vi "Algo test.vi"() -> ()   [LabVIEW 2017]
uses:
  <vilib>/vision/Image Controls.llb/IMAQ Image.ctl
  File/Control/Folder Format.ctl
  File/Control/File Format.ctl
  File/Control/Parent path.ctl
  Toolbox/Control/CVT Action.ctl
  Toolbox/Control/CVT name.vi
  SubVI/File/Section and key name.vi
  <vilib>/vision/NI_Vision_Development_Module.lvlib
  <vilib>/vision/driver/NI_Vision_Acquisition_Software.lvlib
  <vilib>/userdefined/High Color/IMAQdx.ctl
  Toolbox/Toolbox.lvlib
  File/File.lvlib
panel:
  out "Excel copy_Gap inv":sgl[](array[numeric])
  out "Excel copy_Ering inv":dbl[](array[numeric])
  out "Excel copy_Gap":sgl[](array[numeric])
  out "Excel copy_Ering":dbl[](array[numeric])
  out "ERing 4":sgl[](array[numeric]) format="%.3g"
  out "ERing 3":sgl[](array[numeric]) format="%.3g"
  out "ERing 2":sgl[](array[numeric]) format="%.3g"
  out "ERing 1":sgl[](array[numeric]) format="%.3g"
  out "Row1":sgl[](array[numeric]) format="%.3g"
  out "Row2":sgl[](array[numeric]) format="%#.3g"
  out "Row3":sgl[](array[numeric]) format="%#.3g"
  out "Row4":sgl[](array[numeric]) format="%.3g"
  out "Row Match":bool[](array[boolean])
  out "Row time":u32[](array[numeric])
  in  "File Path 2":path
  out "Image":T1(plugin-control)
  out "error out":errorcluster
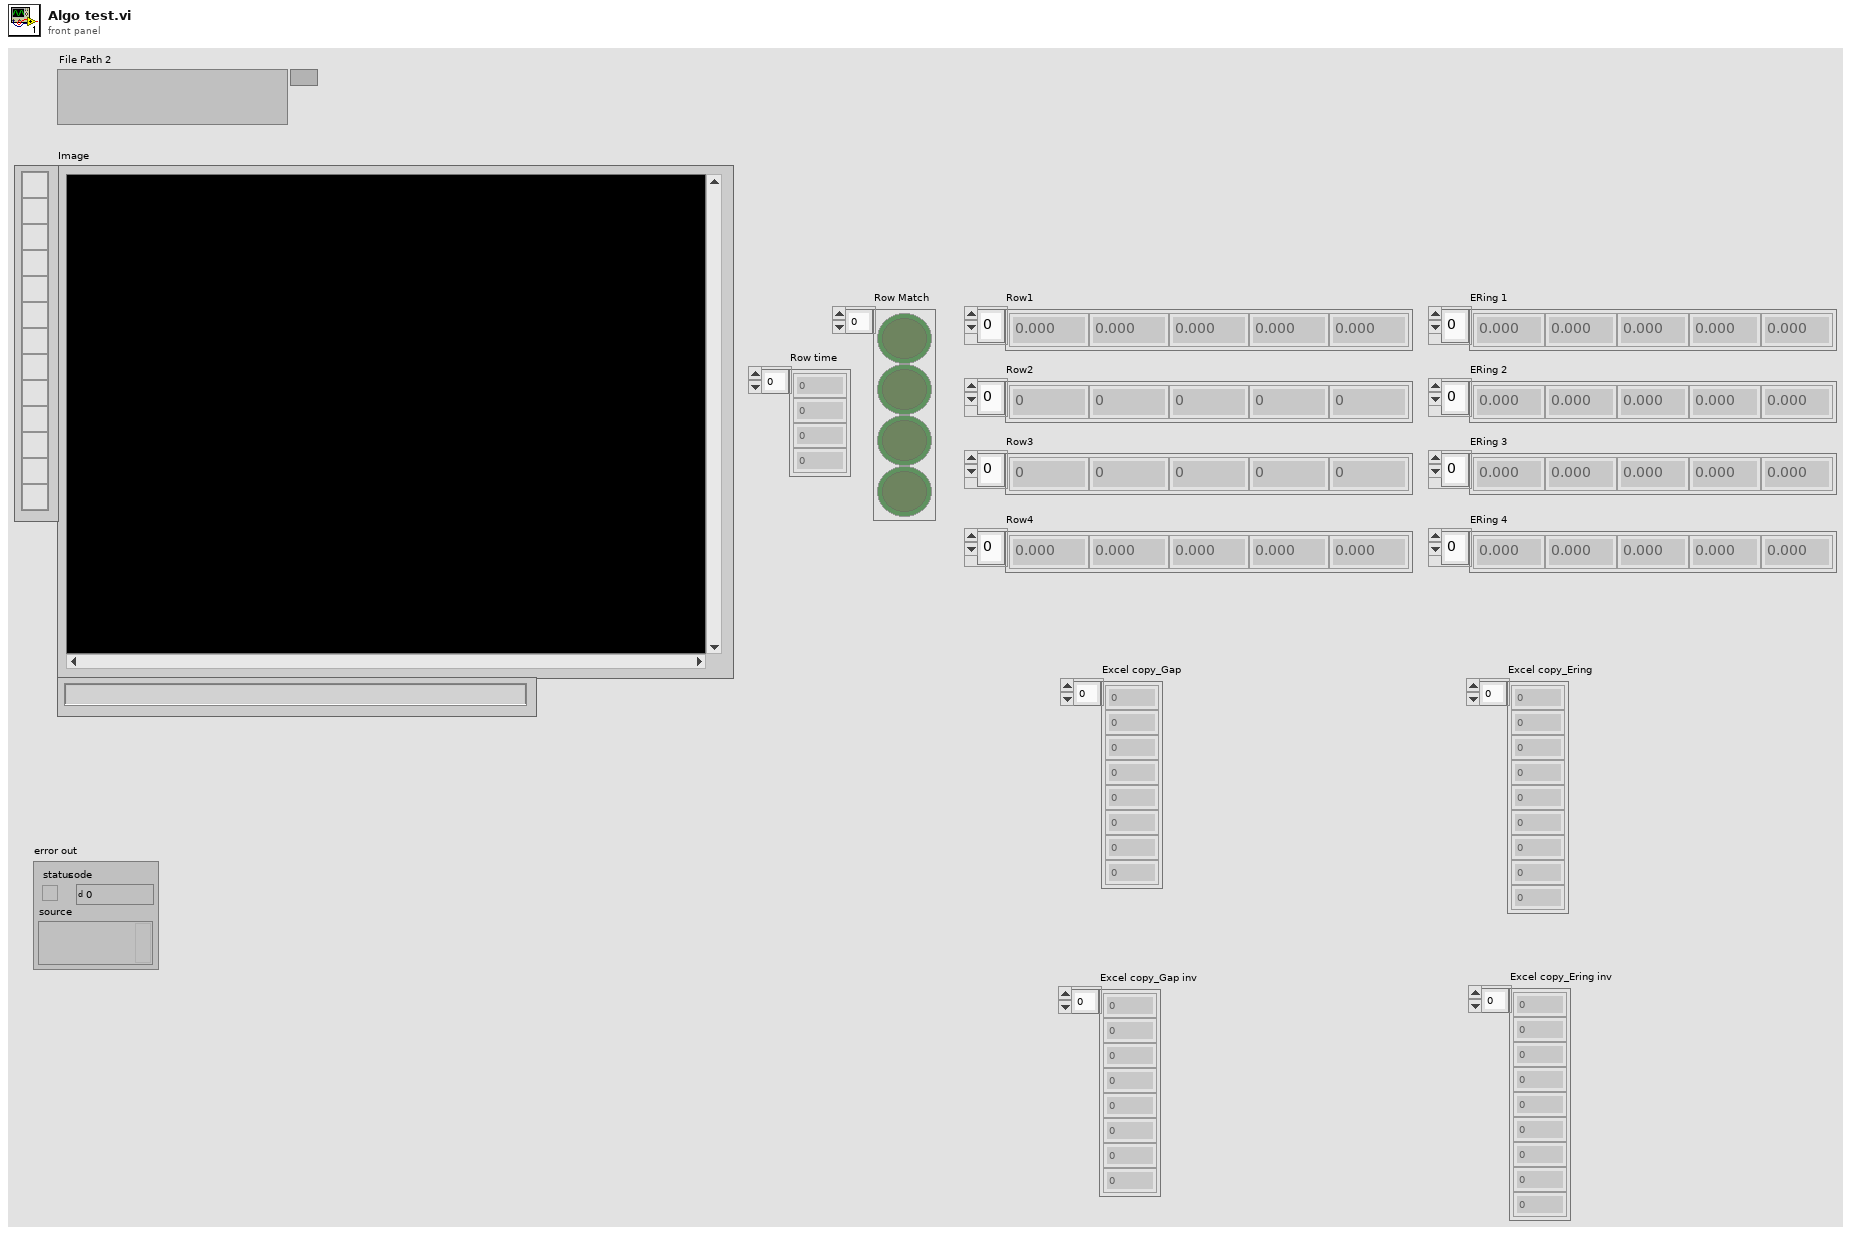
[diagram p1: front panel]
types:
  T1 = typedef "IMAQ Image.ctl" = refnum<image>
  T2 = cluster{"State":string, "snap Image":T1, "Template":T1, "Calibration":T1, "Row1 result":cluster{"Fitted Circle Ering":cluster{"Center (Pixels)":cluster{"X":sgl, "Y":sgl}, "Radius (Pixels)":dbl, "Center (Real-World)":cluster{"X":sgl, "Y":sgl}, "Radius (Real-World)":dbl, "Roundness (Real-World)":dbl, "Average Strength":dbl, "Average SNR (dB)":dbl}, "Fitted Circle Center":cluster{"Center (Pixels)":cluster{"X":sgl, "Y":sgl}, "Radius (Pixels)":dbl, "Center (Real-World)":cluster{"X":sgl, "Y":sgl}, "Radius (Real-World)":dbl, "Roundness (Real-World)":dbl, "Average Strength":dbl, "Average SNR (dB)":dbl}}[], "Row2 result":cluster{"Fitted Circle Ering":cluster{"Center (Pixels)":cluster{"X":sgl, "Y":sgl}, "Radius (Pixels)":dbl, "Center (Real-World)":cluster{"X":sgl, "Y":sgl}, "Radius (Real-World)":dbl, "Roundness (Real-World)":dbl, "Average Strength":dbl, "Average SNR (dB)":dbl}, "Fitted Circle Center":cluster{"Center (Pixels)":cluster{"X":sgl, "Y":sgl}, "Radius (Pixels)":dbl, "Center (Real-World)":cluster{"X":sgl, "Y":sgl}, "Radius (Real-World)":dbl, "Roundness (Real-World)":dbl, "Average Strength":dbl, "Average SNR (dB)":dbl}}[], "Row3 result":cluster{"Fitted Circle Ering":cluster{"Center (Pixels)":cluster{"X":sgl, "Y":sgl}, "Radius (Pixels)":dbl, "Center (Real-World)":cluster{"X":sgl, "Y":sgl}, "Radius (Real-World)":dbl, "Roundness (Real-World)":dbl, "Average Strength":dbl, "Average SNR (dB)":dbl}, "Fitted Circle Center":cluster{"Center (Pixels)":cluster{"X":sgl, "Y":sgl}, "Radius (Pixels)":dbl, "Center (Real-World)":cluster{"X":sgl, "Y":sgl}, "Radius (Real-World)":dbl, "Roundness (Real-World)":dbl, "Average Strength":dbl, "Average SNR (dB)":dbl}}[], "Row4 result":cluster{"Fitted Circle Ering":cluster{"Center (Pixels)":cluster{"X":sgl, "Y":sgl}, "Radius (Pixels)":dbl, "Center (Real-World)":cluster{"X":sgl, "Y":sgl}, "Radius (Real-World)":dbl, "Roundness (Real-World)":dbl, "Average Strength":dbl, "Average SNR (dB)":dbl}, "Fitted Circle Center":cluster{"Center (Pixels)":cluster{"X":sgl, "Y":sgl}, "Radius (Pixels)":dbl, "Center (Real-World)":cluster{"X":sgl, "Y":sgl}, "Radius (Real-World)":dbl, "Roundness (Real-World)":dbl, "Average Strength":dbl, "Average SNR (dB)":dbl}}[]}
  T3 = typedef "File.lvlib/Parent path.ctl" = enum16{"Project", "Setting", "Log"}
  T4 = typedef "File.lvlib/File Format.ctl" = enum16{"None", "File Date", "File Time"}
  T5 = typedef "File.lvlib/Folder Format.ctl" = enum16{"None", "Folder Date", "Folder/Date"}
  T6 = typedef "IMAQdx.ctl" = refnum<k21>
  T7 = typedef "ROI Descriptor" = cluster{"Global Rectangle":i32[], "Contours":cluster{"ID":enum32{"External", "Internal"}, "Type":u32, "Coordinates":i32[]}[]}
  T8 = typedef "Toolbox.lvlib/CVT Action.ctl" = enum16{"Set", "Replace", "Get", "Check", "Delete", "Delete All"}
  T9 = cluster{"Fitted Circle Ering":cluster{"Center (Pixels)":cluster{"X":sgl, "Y":sgl}, "Radius (Pixels)":dbl, "Center (Real-World)":cluster{"X":sgl, "Y":sgl}, "Radius (Real-World)":dbl, "Roundness (Real-World)":dbl, "Average Strength":dbl, "Average SNR (dB)":dbl}, "Fitted Circle Center":cluster{"Center (Pixels)":cluster{"X":sgl, "Y":sgl}, "Radius (Pixels)":dbl, "Center (Real-World)":cluster{"X":sgl, "Y":sgl}, "Radius (Real-World)":dbl, "Roundness (Real-World)":dbl, "Average Strength":dbl, "Average SNR (dB)":dbl}}[]
  T10 = cluster{"Fitted Circle Ering":cluster{"Center (Pixels)":cluster{"X":sgl, "Y":sgl}, "Radius (Pixels)":dbl, "Center (Real-World)":cluster{"X":sgl, "Y":sgl}, "Radius (Real-World)":dbl, "Roundness (Real-World)":dbl, "Average Strength":dbl, "Average SNR (dB)":dbl}, "Fitted Circle Center":cluster{"Center (Pixels)":cluster{"X":sgl, "Y":sgl}, "Radius (Pixels)":dbl, "Center (Real-World)":cluster{"X":sgl, "Y":sgl}, "Radius (Real-World)":dbl, "Roundness (Real-World)":dbl, "Average Strength":dbl, "Average SNR (dB)":dbl}}[][]
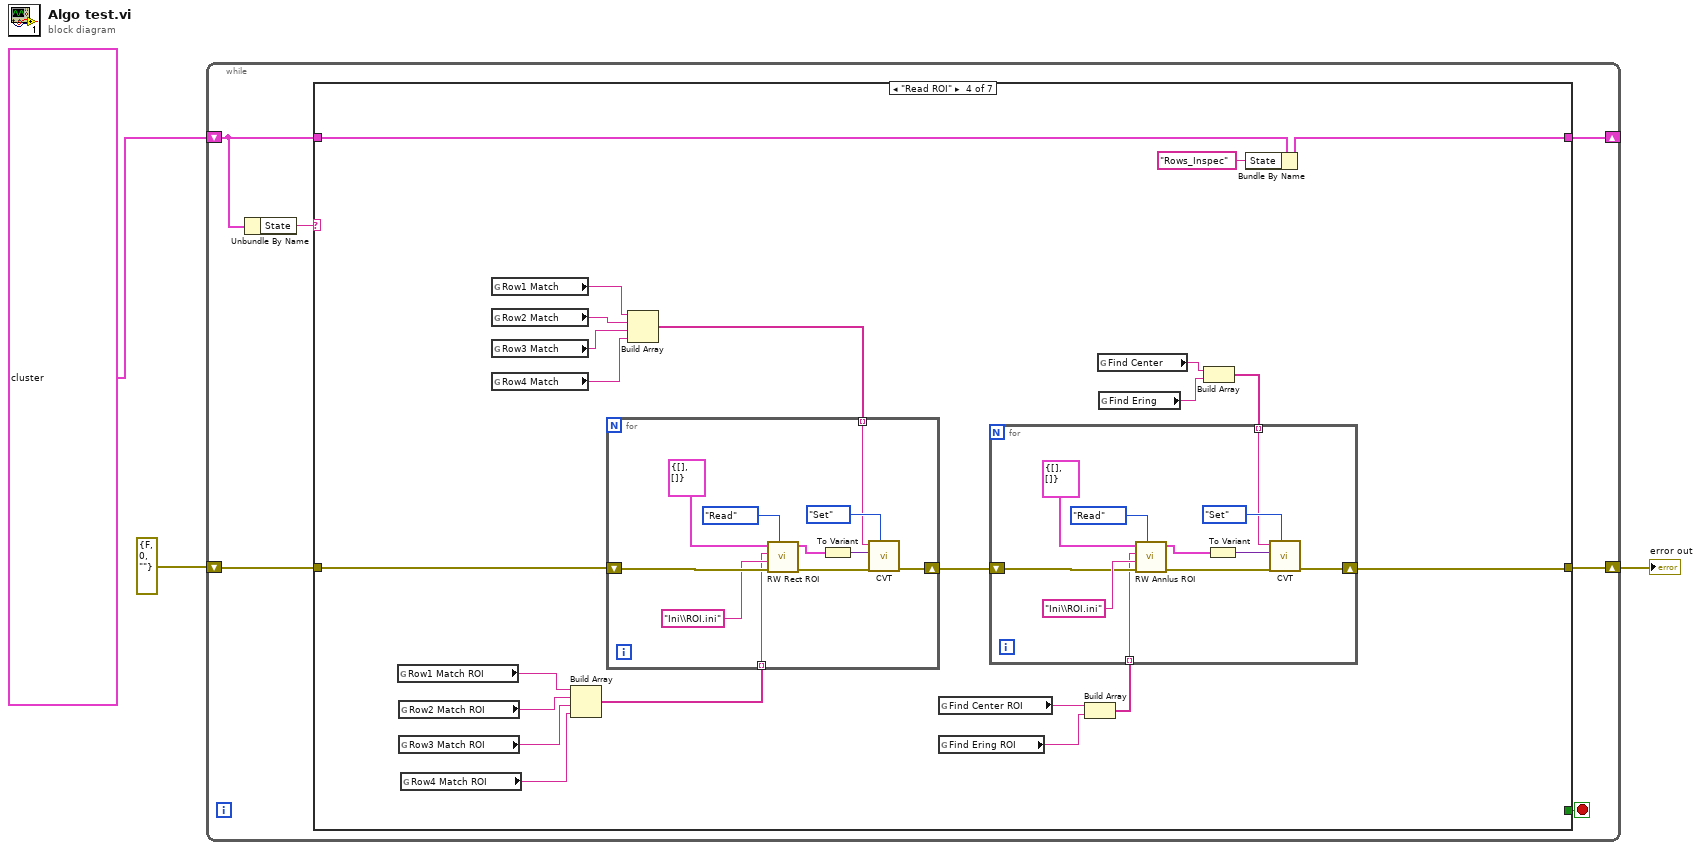
[diagram p0: block diagram]
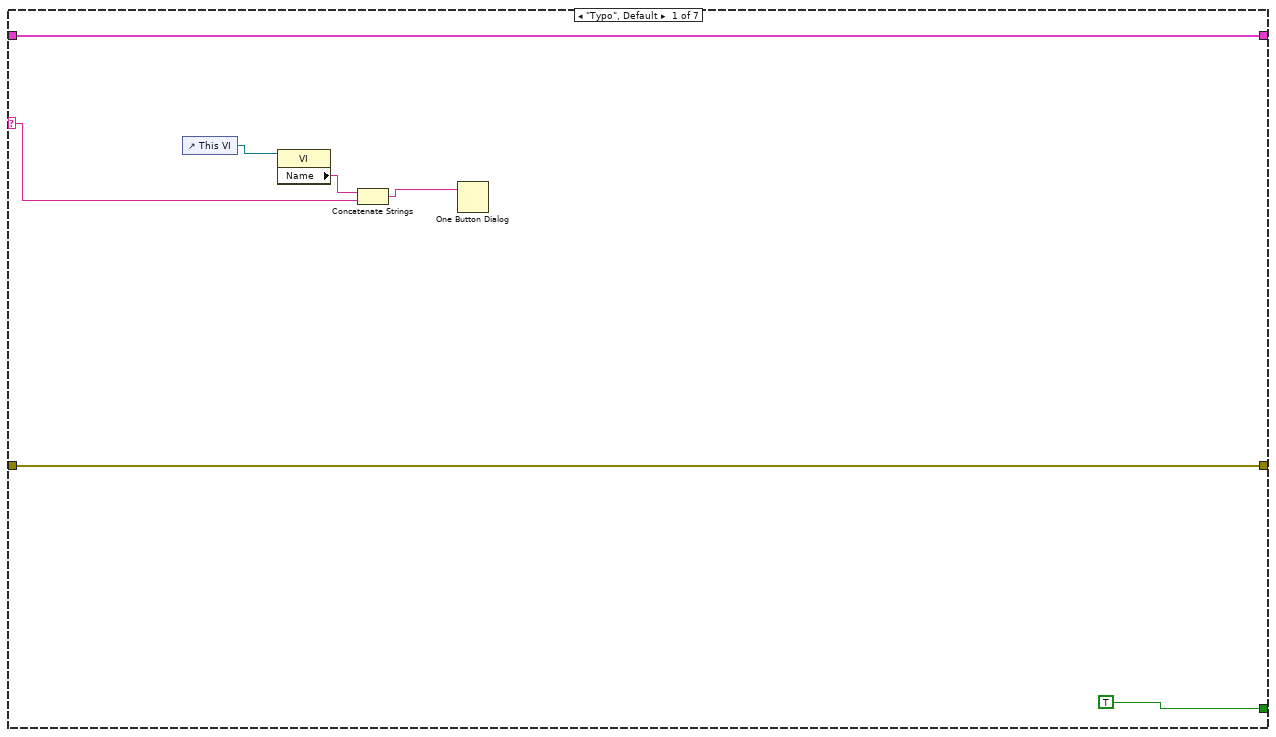
[diagram p2: hidden frame]
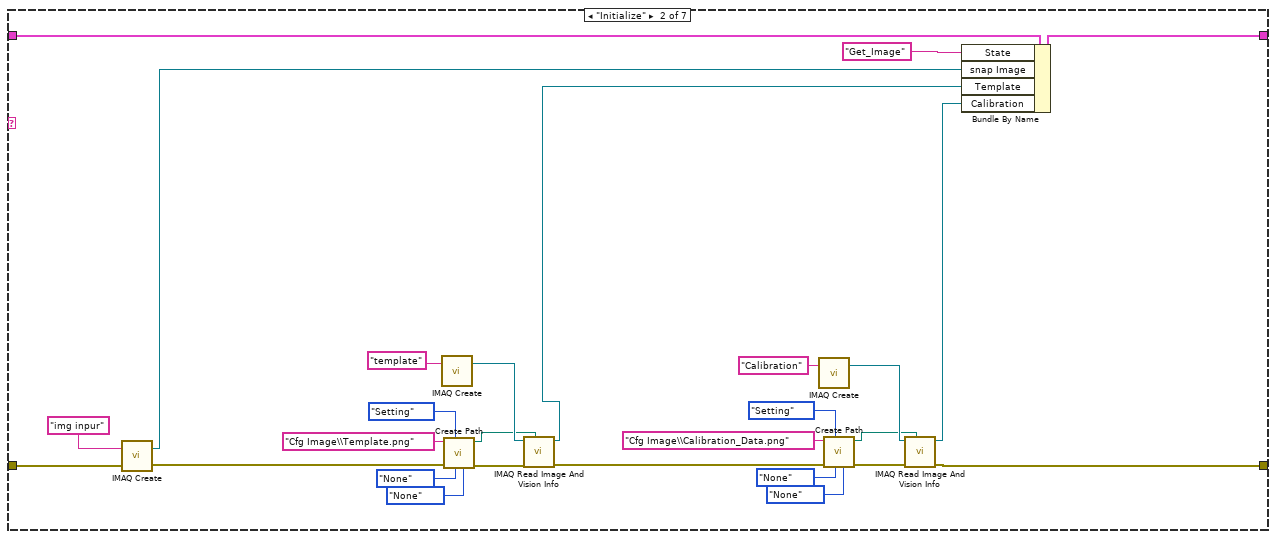
[diagram p3: hidden frame]
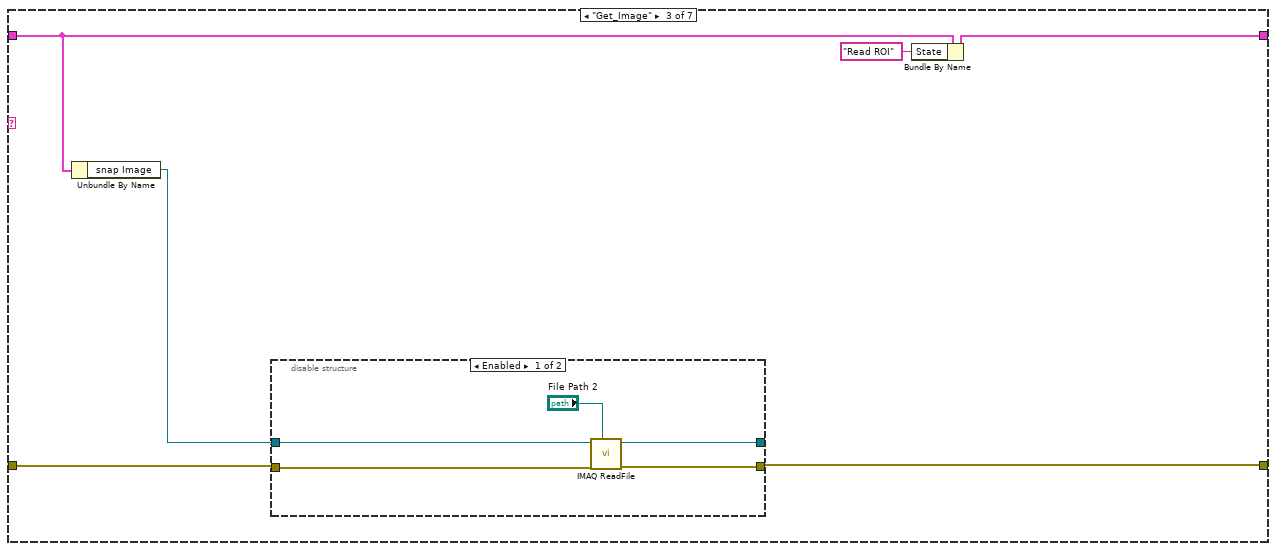
[diagram p4: hidden frame]
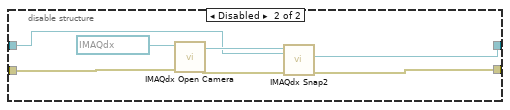
[diagram p5: hidden frame]
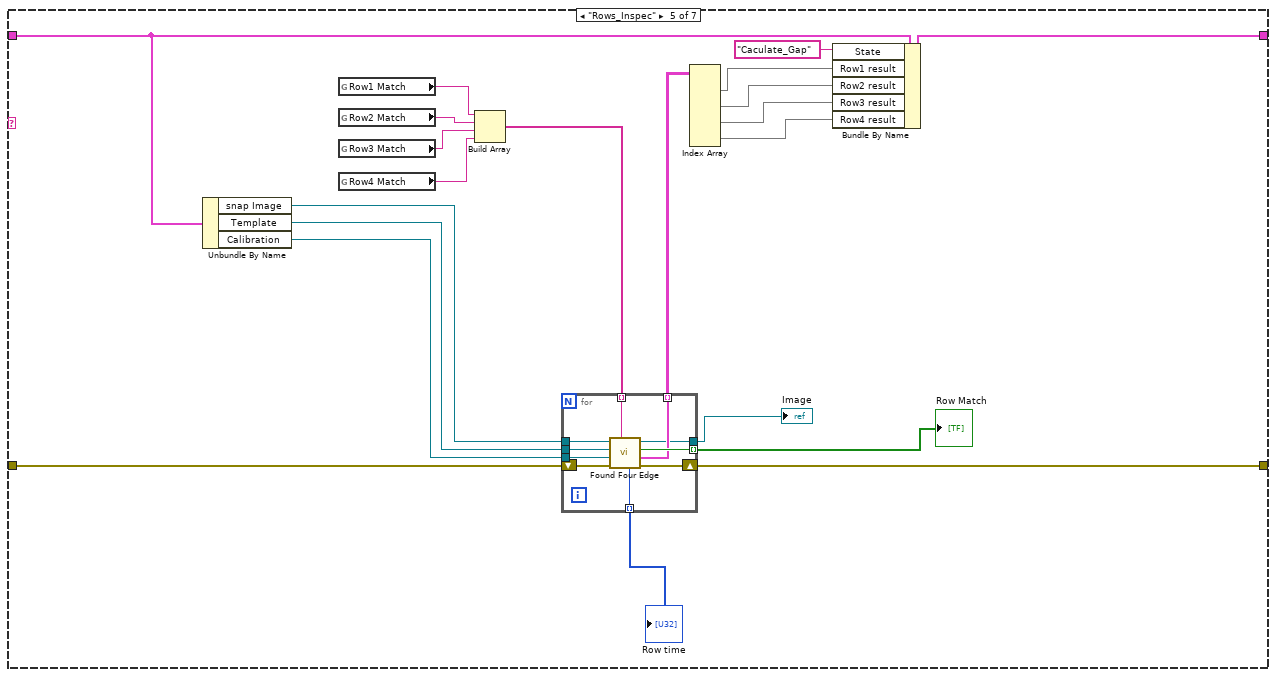
[diagram p6: hidden frame]
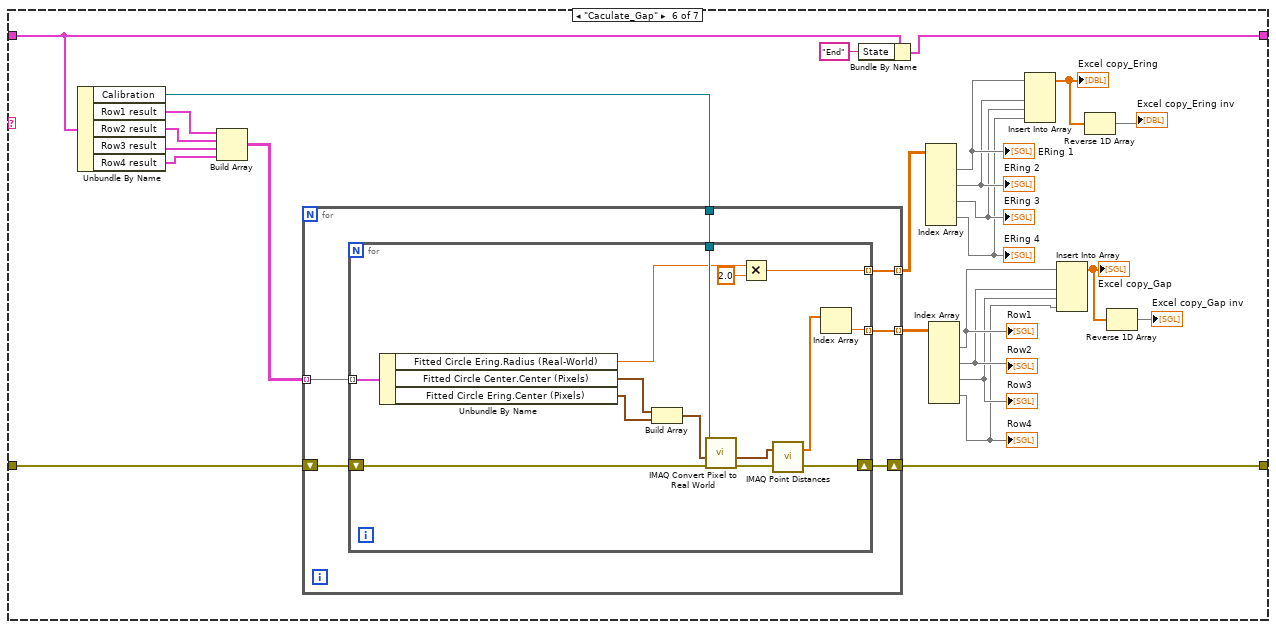
[diagram p7: hidden frame]
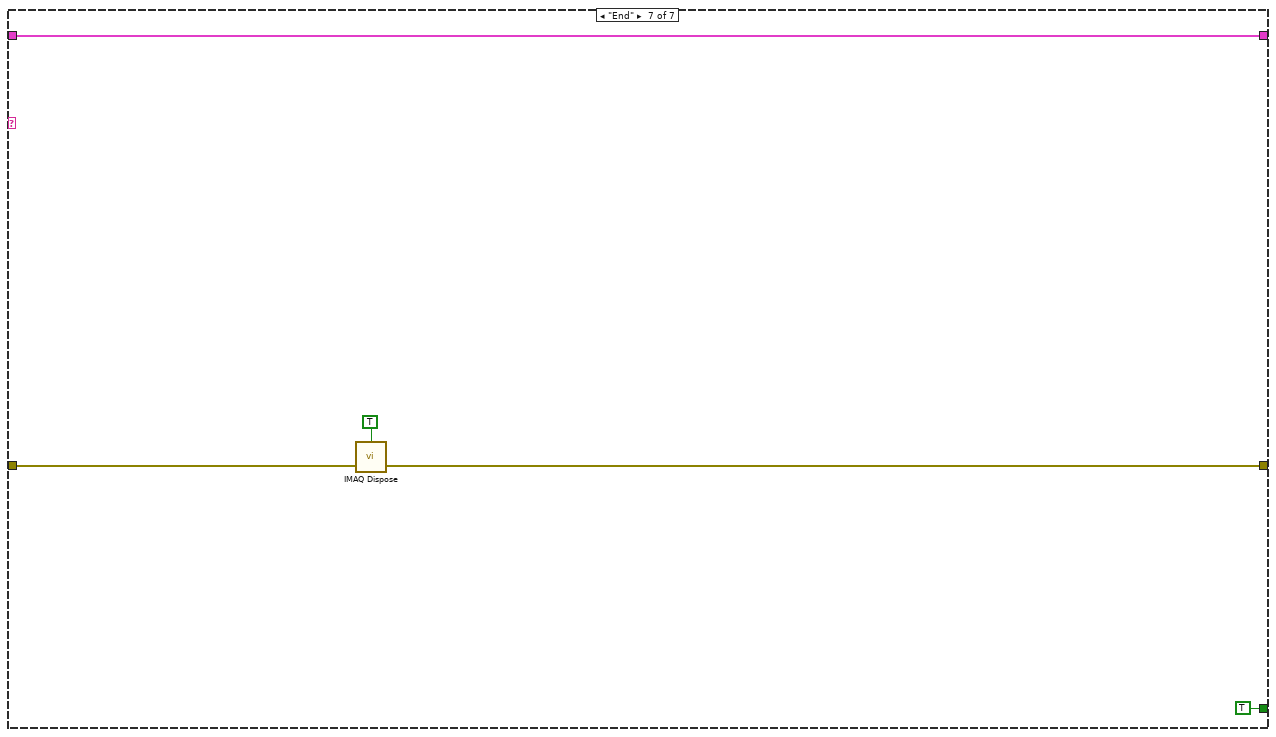
[diagram p8: hidden frame]
diagram:
  n1 = while {
    shift-right: [w8] -> _
    shift-left: T2 {"State"="Initialize", "snap Image"=refnum, "Template"=refnum, "Calibration"=refnum, "Row1 result"=[], "Row2 result"=[], "Row3 result"=[], "Row4 result"=[]} -> [w7]
    shift-right: [w5] -> w1
    shift-left: errorcluster {"status"=FALSE, "code"=0, "source"=""} ("error in (no error)") -> [w6]
    stop <- w4 stop-if-true
    n2 = Unbundle By Name(w7) -> ("State"=w9:string)
    n3 = case shown="\"Read ROI\"" w9 {
      selector: w9 -> [w13 _ _ _ _ _ _]
      tunnel: [w16 w42 w45 w63 w113 w138 w185] -> w8
      tunnel: w7 -> [w16 w43 w48 w83 w124 w159 w185]
      tunnel: w6 -> [w11 w36 w49 w65 w126 w161 w184]
      tunnel: [w11 w35 w46 w64 w125 w160 w183] -> w5
      tunnel: [TRUE _ _ _ _ _ TRUE] -> w4
      frame "Typo", Default {
        n4 = control-ref of="This VI"() -> (w15:refnum<vi>)
        n5 = property class="VI"(reference=w15) -> ("Name"=w14:string)  [unwired: 1 in, 2 out]
        n6 = Concatenate Strings(w14, w13) -> (w12:string)
        n7 = One Button Dialog(message=w12) -> ()  [unwired: 1 in, 1 out]
      }
      frame "Initialize" {
        n8 = call "IMAQ Create"("Image Name"="img inpur", "error in (no error)"=w36) -> ("New Image"=w33:T1, "error out"=w30:errorcluster)  [unwired: 3 in]
        n9 = call "IMAQ Create"("Image Name"="template") -> ("New Image"=w40:T1)  [unwired: 4 in, 1 out]
        n10 = call "Create Path.vi"("File Format"=File_Format."None", "Folder Format"=Folder_Format."None", "Parent path"=Parent_path."Setting", "error in (no error)"=w30, "Directory"="Cfg Image\\Template.png") -> ("error out"=w29:errorcluster, "Path"=w24:path)  [unwired: 5 in]
        n11 = call "IMAQ Read Image And Vision Info"("File Path"=w24, "error in (no error)"=w29, "Image"=w40) -> ("error out"=w19:errorcluster, "Image Out"=w32:T1)  [unwired: 6 in, 1 out]
        n12 = call "IMAQ Create"("Image Name"="Calibration") -> ("New Image"=w37:T1)  [unwired: 4 in, 1 out]
        n13 = call "Create Path.vi"("File Format"=File_Format."None", "Folder Format"=Folder_Format."None", "Parent path"=Parent_path."Setting", "error in (no error)"=w19, "Directory"="Cfg Image\\Calibration_Data.png") -> ("error out"=w18:errorcluster, "Path"=w17:path)  [unwired: 5 in]
        n14 = call "IMAQ Read Image And Vision Info"("File Path"=w17, "error in (no error)"=w18, "Image"=w37) -> ("error out"=w35:errorcluster, "Image Out"=w31:T1)  [unwired: 6 in, 1 out]
        n15 = Bundle By Name(cluster=w43, "State"="Get_Image", "snap Image"=w33, "Template"=w32, "Calibration"=w31) -> (w42:T2)
      }
      frame "Get_Image" {
        n16 = Unbundle By Name(w48) -> ("snap Image"=w47:T1)
        n17 = disable-structure shown="Enabled" {
          disable-tunnel: [w53 w56] -> _
          disable-tunnel: [w52 w59] -> w46
          disable-tunnel: w47 -> [w51 w57]
          disable-tunnel: w49 -> [w50 w55]
          frame Enabled {
            n18 = call "IMAQ ReadFile"("File Path"="File Path 2", "error in (no error)"=w50, "Image"=w51) -> ("error out"=w52:errorcluster, "Image Out"=w53:T1)  [unwired: 4 in, 3 out]
          }
          frame Disabled {
            n19 = call <vilib>:"IMAQdx Open Camera.vi"("error in"=w55, "Session In"=T6 "cam004") -> ("error out"=w60:errorcluster, "Session Out"=w61:T6)  [unwired: 8 in]
            n20 = call <vilib>:"IMAQdx Snap2.vi"("error in"=w60, "Image In"=w57, "Session In"=w61) -> ("error out"=w59:errorcluster, "Image Out"=w56:T1)  [unwired: 6 in, 1 out]
          }
        }
        n21 = Bundle By Name(cluster=w48, "State"="Read ROI") -> (w45:T2)
      }
      frame "Read ROI" {
        n22 = global read "Section and key name.vi" "Row1 Match ROI"() -> (w67:string)
        n23 = global read "Section and key name.vi" "Row2 Match ROI"() -> (w68:string)
        n24 = global read "Section and key name.vi" "Row3 Match ROI"() -> (w69:string)
        n25 = global read "Section and key name.vi" "Row4 Match ROI"() -> (w70:string)
        n26 = global read "CVT name.vi" "Row1 Match"() -> (w72:string)
        n27 = global read "CVT name.vi" "Row2 Match"() -> (w73:string)
        n28 = global read "CVT name.vi" "Row3 Match"() -> (w74:string)
        n29 = global read "CVT name.vi" "Row4 Match"() -> (w75:string)
        n30 = Build Array(w67, w68, w69, w70) -> (w66:string[])
        n31 = Build Array(w72, w73, w74, w75) -> (w71:string[])
        n32 = for {
          shift-right: [w86] -> w82
          shift-left: w65 -> [w91]
          tunnel: w71 -> [w85] mode=indexing
          tunnel: w66 -> [w84] mode=indexing
          n33 = call "RW Rect ROI.vi"("Read/Write"=enum16{"Read", "Write"}."Read", "error in (no error)"=w91, "directory Path"="Ini\\ROI.ini", "section"=w84, "ROI Descriptor"=T7 {"Global Rectangle"=[], "Contours"=[]}) -> ("error out"=w90:errorcluster, "ROI Descriptor Out"=w89:T7)  [unwired: 5 in]
          n34 = To Variant(anything=w89) -> (Variant=w88:variant)
          n35 = call "CVT.vi"("Action"=CVT_Action."Set", "error in (no error)"=w90, "Value in"=w88, "Key"=w85) -> ("error out"=w86:errorcluster)  [unwired: 5 in, 2 out]
        }
        n36 = global read "Section and key name.vi" "Find Center ROI"() -> (w78:string)
        n37 = global read "Section and key name.vi" "Find Ering ROI"() -> (w77:string)
        n38 = Build Array(w78, w77) -> (w76:string[])
        n39 = global read "CVT name.vi" "Find Center"() -> (w80:string)
        n40 = global read "CVT name.vi" "Find Ering"() -> (w81:string)
        n41 = Build Array(w80, w81) -> (w79:string[])
        n42 = for {
          shift-right: [w99] -> w64
          shift-left: w82 -> [w97]
          tunnel: w79 -> [w95] mode=indexing
          tunnel: w76 -> [w96] mode=indexing
          n43 = call "RW Annlus ROI.vi"("Read/Write"=enum16{"Read", "Write"}."Read", "error in (no error)"=w97, "directory Path"="Ini\\ROI.ini", "section"=w96, "ROI Descriptor"=T7 {"Global Rectangle"=[], "Contours"=[]}) -> ("error out"=w102:errorcluster, "ROI Descriptor Out"=w101:T7)  [unwired: 5 in]
          n44 = To Variant(anything=w101) -> (Variant=w100:variant)
          n45 = call "CVT.vi"("Action"=CVT_Action."Set", "error in (no error)"=w102, "Value in"=w100, "Key"=w95) -> ("error out"=w99:errorcluster)  [unwired: 5 in, 2 out]
        }
        n46 = Bundle By Name(cluster=w83, "State"="Rows_Inspec") -> (w63:T2)
      }
      frame "Rows_Inspec" {
        n47 = Unbundle By Name(w124) -> ("snap Image"=w123:T1, "Template"=w122:T1, "Calibration"=w121:T1)
        n48 = global read "CVT name.vi" "Row1 Match"() -> (w116:string)
        n49 = global read "CVT name.vi" "Row2 Match"() -> (w117:string)
        n50 = global read "CVT name.vi" "Row3 Match"() -> (w118:string)
        n51 = global read "CVT name.vi" "Row4 Match"() -> (w119:string)
        n52 = Build Array(w116, w117, w118, w119) -> (w115:string[])
        n53 = for {
          tunnel: w123 -> [w134]
          tunnel: w122 -> [w133]
          tunnel: w121 -> [w132]
          shift-right: [w135] -> w125
          shift-left: w126 -> [w136]
          tunnel: [w131] -> w120 mode=indexing
          tunnel: w115 -> [w130] mode=indexing
          tunnel: [w129] -> w114 mode=indexing
          tunnel: [w128] -> w110 mode=indexing
          tunnel: [w127] -> w111
          n54 = call "Found Four Edge.vi"("Row ROI Name"=w130, "error in"=w136, "Calibration"=w132, "Template"=w133, "Image In"=w134) -> ("error out"=w135:errorcluster, "Array of Fitting"=w128:T9, "Match?"=w129:bool, "Image out"=w127:T1, "Elapsed time(ms)"=w131:u32)  [unwired: 2 in]
        }
        "Row time" <- w120
        "Row Match" <- w114
        "Image" <- w111
        n55 = Index Array(array=w110) -> (element #1=w109:T9, element #2=w108:T9, element #3=w107:T9, element #4=w106:T9)  [unwired: 8 in]
        n56 = Bundle By Name(cluster=w124, "State"="Caculate_Gap", "Row1 result"=w109, "Row2 result"=w108, "Row3 result"=w107, "Row4 result"=w106) -> (w113:T2)
      }
      frame "Caculate_Gap" {
        n57 = Unbundle By Name(w159) -> ("Calibration"=w151:T1, "Row1 result"=w158:T9, "Row2 result"=w157:T9, "Row3 result"=w156:T9, "Row4 result"=w155:T9)
        n58 = Build Array(w158, w157, w156, w155) -> (w154:T10)
        n59 = for {
          shift-right: [w166] -> w160
          shift-left: w161 -> [w167]
          tunnel: w154 -> [w165] mode=indexing
          tunnel: [w164] -> w152 mode=indexing
          tunnel: [w163] -> w153 mode=indexing
          tunnel: w151 -> [w162]
          n60 = for {
            tunnel: [w170] -> w164 mode=indexing
            tunnel: [w172] -> w163 mode=indexing
            shift-right: [w176] -> w166
            shift-left: w167 -> [w181]
            tunnel: w165 -> [w174] mode=indexing
            tunnel: w162 -> [w171]
            n61 = Unbundle By Name(w174) -> ("Fitted Circle Ering.Radius (Real-World)"=w169:dbl, "Fitted Circle Center.Center (Pixels)"=w180:cluster{"X":sgl, "Y":sgl}, "Fitted Circle Ering.Center (Pixels)"=w179:cluster{"X":sgl, "Y":sgl})
            n62 = Build Array(w180, w179) -> (w175:cluster{"X":sgl, "Y":sgl}[])
            n63 = call "IMAQ Convert Pixel to Real World"("error in (no error)"=w181, "Array of Pixel Coordinates"=w175, "Calibrated Image"=w171) -> ("error out"=w178:errorcluster, "Array of Real World Coordinates"=w177:cluster{"X":sgl, "Y":sgl}[])  [unwired: 3 in, 4 out]
            n64 = Multiply(x=w169, y=2.0) -> (x*y=w170:dbl)
            n65 = call "IMAQ Point Distances"("Points"=w177, "error in (no error)"=w178) -> ("Distances"=w173:sgl[], "error out"=w176:errorcluster)  [unwired: 3 in]
            n66 = Index Array(array=w173) -> (element=w172:sgl)  [unwired: 1 in]
          }
        }
        n67 = Bundle By Name(cluster=w159, "State"="End") -> (w138:T2)
        n68 = Index Array(array=w152) -> (element #1=w150:dbl[], element #2=w149:dbl[], element #3=w148:dbl[], element #4=w147:dbl[])  [unwired: 8 in]
        "ERing 1" <- w150
        "ERing 2" <- w149
        "ERing 3" <- w148
        "ERing 4" <- w147
        n69 = Index Array(array=w153) -> (element #1=w146:sgl[], element #2=w145:sgl[], element #3=w144:sgl[], element #4=w143:sgl[])  [unwired: 8 in]
        "Row4" <- w143
        "Row3" <- w144
        "Row2" <- w145
        "Row1" <- w146
        n70 = Insert Into Array(array=w150, new element #1=w149, new element #2=w148, new element #3=w147) -> (w142:dbl[])  [unwired: 1 in]
        "Excel copy_Ering" <- w142
        n71 = Insert Into Array(array=w146, new element #1=w145, new element #2=w144, new element #3=w143) -> (w139:sgl[])  [unwired: 1 in]
        "Excel copy_Gap" <- w139
        n72 = Reverse 1D Array(array=w142) -> (reversed array=→"Excel copy_Ering inv":dbl[])
        n73 = Reverse 1D Array(array=w139) -> (reversed array=→"Excel copy_Gap inv":sgl[])
      }
      frame "End" {
        n74 = call "IMAQ Dispose"("All Images? (No)"=TRUE, "error in (no error)"=w184) -> ("error out"=w183:errorcluster)  [unwired: 4 in]
      }
    }
  }
  "error out" <- w1
